vi "Load Help File.vi"(8 "error in":errorcluster, 9 "HTML File to Load":string, 11 "Browser":refnum<k7>(container)) -> (0 "error out":errorcluster)   [LabVIEW 2026, in "SystemMonitor System Explorer.lvlib"]
doc: "Loads the specified HTML page from the CHM into the browser"
uses:
  SystemMonitor System Explorer.lvlib
  <vilib>/Utility/LVLibp/NI_PackedLibraryUtility.lvlib
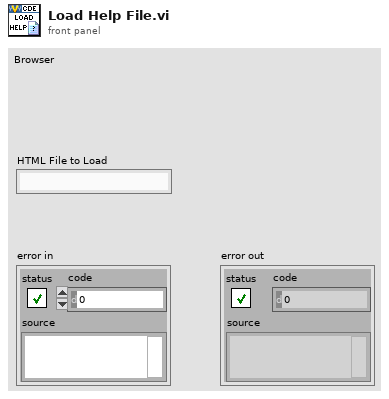
[diagram p1: front panel]
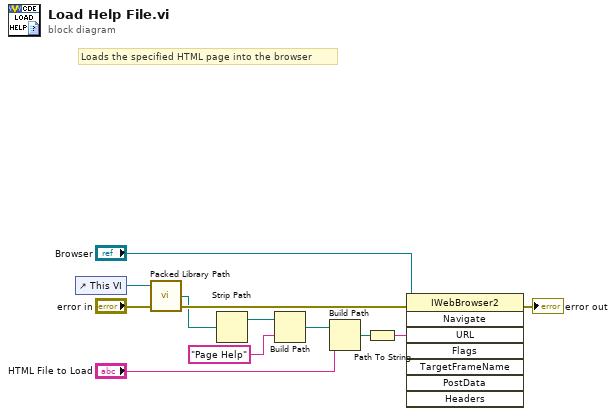
[diagram p0: block diagram]
diagram:
  # "Loads the specified HTML page into the browser"
  n1 = control-ref of="This VI"() -> (w11:refnum<vi>)
  n2 = call <vilib>:"Packed Library Path.vi"("error in (no error)"="error in", "vi reference"=w11) -> ("error out"=w7:errorcluster, "packed library path"=w5:path)  [unwired: 1 in, 1 out]
  n3 = Strip Path(path=w5) -> (stripped path=w9:path)  [unwired: 1 out]
  n4 = Build Path(base path=w9, name or relative path="Page Help" ("string")) -> (appended path=w2:path)
  n5 = Build Path(base path=w2, name or relative path="HTML File to Load") -> (appended path=w1:path)
  n6 = Path To String(path=w1) -> (string=w6:string)
  n7 = invoke class="IWebBrowser2" method="Navigate"(reference="Browser", error in=w7, "URL"=w6) -> (error out=→"error out":errorcluster)  [unwired: 5 in, 7 out]
